vi "initialize Session Data.vi"(0 "OBJ - Session in":refnum<class "System Log.lvclass">, 11 "error in":errorcluster) -> (4 "OBJ - Session out":refnum<class "System Log.lvclass">, 15 "error out":errorcluster)   [LabVIEW 2015, in "System Log.lvclass"]
doc: "OVERRIDE VI\nPlaceholder for decendant sessions to initialize and set their default values"
uses:
  System Log.lvclass
  System Log.lvclass/System Log.ctl
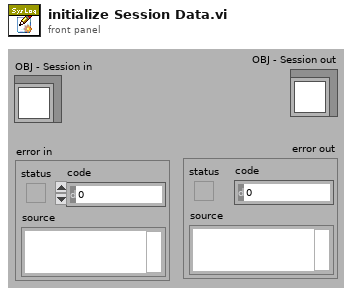
[diagram p1: front panel]
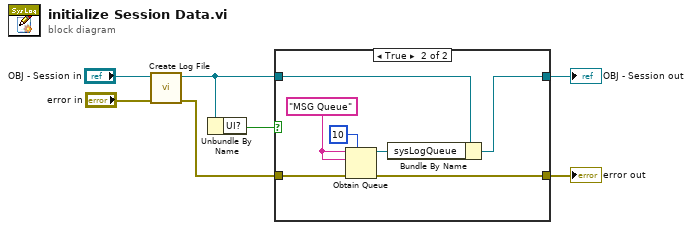
[diagram p0: block diagram]
diagram:
  n1 = call "Create Log File.vi"("error in"="error in", "Sys Log in"="OBJ - Session in") -> ("error out"=w4:errorcluster, "Sys Log out"=w3:refnum<class "System Log.lvclass">)  [unwired: 8 in]
  n2 = Unbundle By Name(w3) -> ("UI?"=w2:bool)
  n3 = case shown="True" w2 {
    tunnel: [w9 w10] -> w5
    tunnel: w4 -> [w8 w16]
    tunnel: w3 -> [w9 w12]
    tunnel: [w8 w11] -> w1
    frame False {
    }
    frame True {
      w14 = "MSG Queue" ("name (unnamed)")
      n4 = Obtain Queue(max queue size (-1, unlimited)=10, name (unnamed)=w14, element data type=w14, error in (no error)=w16) -> (queue out=w13:refnum<queue>, error out=w11:errorcluster)  [unwired: 1 in, 1 out]
      n5 = Bundle By Name(cluster=w12, "sysLogQueue"=w13) -> (w10:refnum<class "System Log.lvclass">)
    }
  }
  "OBJ - Session out" <- w5
  "error out" <- w1
